vi "Pre-Build VI - Run Unit Tests.vi"(8 "error in (no error)":errorcluster) -> (0 "error out":errorcluster, 1 "VIs without test coverage":string[](array[string]), 2 "error type":enum16{"fatal", "non-fatal", "warning"}(ring), 5 "num_passed":i32, 7 "num_tested":i32)   [LabVIEW 2020]
uses:
  <userlib>/_OpenG.lib/array/array.llb/Filter 1D Array (String)__ogtk.vi
panel:
  in  "type specifier VI Refnum (for type only)":refnum<vi>
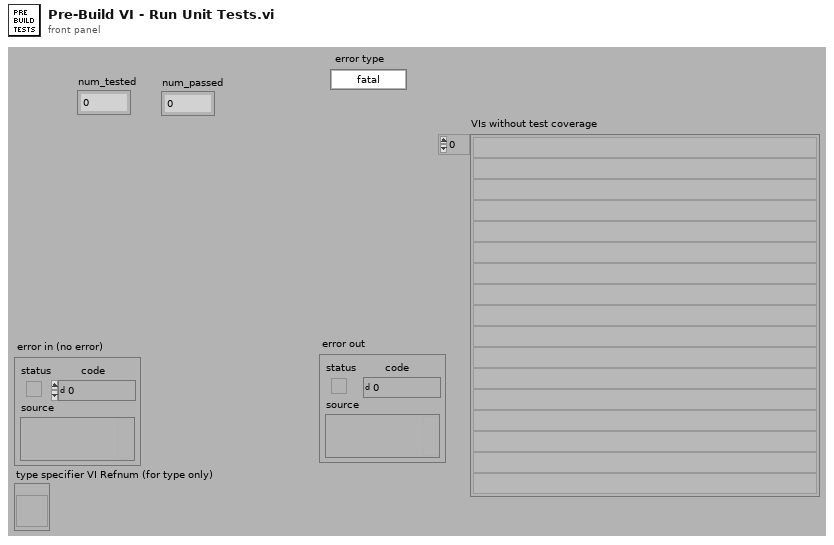
[diagram p1: front panel]
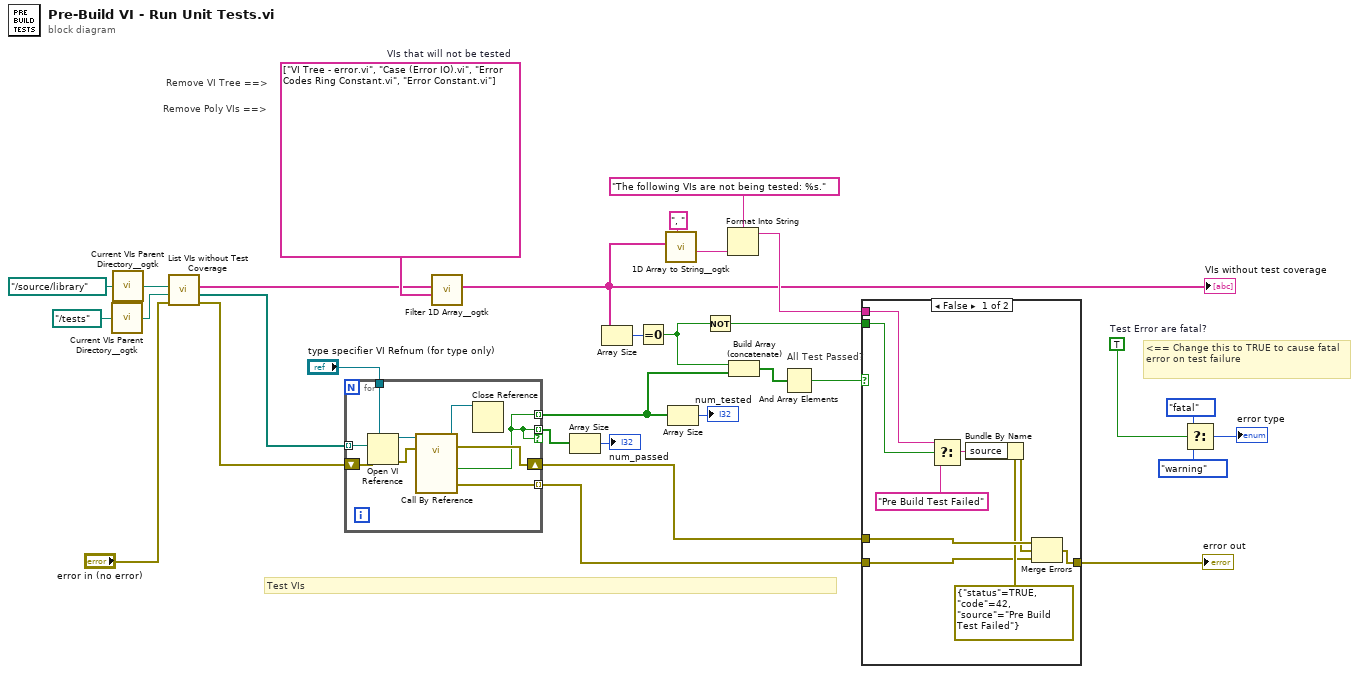
[diagram p0: block diagram]
diagram:
  w18 = TRUE  # Test Error are fatal?
  w29 = string[] ["VI Tree - error.vi", "Case (Error IO).vi", "Error Codes Ring Constant.vi", "Error Constant.vi"]  # VIs that will not be tested
  # "<== Change this to TRUE to cause fatal error on test failure"
  # "Remove Poly VIs ==>"
  # "Remove VI Tree ==>"
  # "All Test Passed?"
  # "Test VIs"
  n1 = call <userlib>:"Current VIs Parent Directory__ogtk.vi"("Relative path (.)"=path "../tests") -> ("Parent Directory (+ Relative)"=w13:path)  [unwired: 4 in]
  n2 = call <userlib>:"Current VIs Parent Directory__ogtk.vi"("Relative path (.)"=path "../source/library") -> ("Parent Directory (+ Relative)"=w22:path)  [unwired: 4 in]
  n3 = call "List VIs without Test Coverage.vi"("error in (no error)"="error in (no error)", "Tests Root"=w13, "Source Root"=w22) -> ("error out"=w9:errorcluster, "Test VIs"=w12:path[], "VIs without test coverage"=w28:string[])  [unwired: 6 in]
  n4 = for {
    tunnel: w12 -> [w40] mode=indexing
    tunnel: "type specifier VI Refnum (for type only)" -> [w39]
    shift-right: [w36] -> w10
    shift-left: w9 -> [w35]
    tunnel: [w32] -> w4 mode=indexing
    tunnel: [w33] -> w8 mode=indexing
    tunnel: [w32] -> w1 mode=indexing if=w32
    n5 = Open VI Reference(type specifier VI Refnum (for type only)=w39, vi path=w40, error in (no error)=w35) -> (vi reference=w38:refnum<vi>, error out=w37:errorcluster)  [unwired: 3 in]
    n6 = call-by-ref "?"(reference=w38, error in=w37) -> (reference out=w34:refnum<vi>, error out=w36:errorcluster, 0:"error out"=w33:errorcluster, "pass"=w32:bool)  [unwired: 10 in]
    n7 = Close Reference(reference=w34) -> ()  [unwired: 1 in, 1 out]
  }
  n8 = call-poly <userlib>:"Filter 1D Array__ogtk.vi"("items to filter"=w29, "array"=w28) -> ("filtered array"=w7:string[])  [unwired: 4 in, 1 out]
  "VIs without test coverage" <- w7
  n9 = Array Size(array=w1) -> (size(s)=→"num_passed":i32)
  n10 = Array Size(array=w7) -> (size(s)=w6:i32)
  n11 = Equal To 0?(x=w6) -> (x = 0?=w5:bool)
  n12 = call <userlib>:"1D Array to String__ogtk.vi"("delimiter (Tab)"=", ", "Array of Strings"=w7) -> ("delimited string"=w26:string)  [unwired: 9 in]
  n13 = Array Size(array=w4) -> (size(s)=→"num_tested":i32)
  n14 = Not(x=w5) -> (.not. x?=w23:bool)
  n15 = Format Into String(format string="The following VIs are not being tested: %s.", w26) -> (resulting string=w24:string)  [unwired: 2 in, 1 out]
  n16 = Build Array (concatenate)(w5, w4) -> (w31:bool[])
  n17 = And Array Elements(Boolean array=w31) -> (logical AND=w30:bool)
  n18 = case shown="False" w30 {
    tunnel: w10 -> [w49 w50]
    tunnel: [w48 w50] -> w20
    tunnel: w23 -> [w47 _]
    tunnel: w24 -> [w46 _]
    tunnel: w8 -> [w41 _]
    frame False {
      n19 = Select(t=w46, s=w47, f="Pre Build Test Failed" ("source")) -> (s? t:f=w44:string)
      n20 = Bundle By Name(cluster=errorcluster {"status"=TRUE, "code"=42, "source"="Pre Build Test Failed"} ("error out"), "source"=w44) -> (w43:errorcluster)
      n21 = Merge Errors(w49, w43, w41) -> (w48:errorcluster)
    }
    frame True {
    }
  }
  "error out" <- w20
  n22 = Select(t=enum16{"fatal", "non-fatal", "warning"}."fatal" ("error type"), s=w18, f=enum16{"fatal", "non-fatal", "warning"}."warning" ("error type")) -> (s? t:f=→"error type":enum16{"fatal", "non-fatal", "warning"})
